vi "Save-Recall Instrument Setup from file.vi"(0 "VISA resource name":refnum<visa-resource-name>, 5 "Action (0:Save Instrument Setup)":u16(ring) items=["Save Instrument Setup", "Recall Instrument Setup"], 9 "Timeout (10000)":u32=10000, 11 "error in (no error)":errorcluster, 12 "Path":string, 13 "Filename (PANEL.SET)":string="PANEL.SET") -> (4 "VISA resource name out":refnum<visa-resource-name>, 15 "error out":errorcluster)   [LabVIEW 2021, in "Siglent SDS 1000 2000 Series.lvlib"]
doc: "Stores or recalls the current state of your instrument to/from a file on the scope's harddrive.\n\nNote:\nTo save or recall panel setups to one of the \"internal\" non-volatile memories, use the VI \"Save-Recall Setup from Device\""
uses:
  <instrlib>/Siglent SDS 1000 2000 Series/Siglent SDS 1000 2000 Series.lvlib
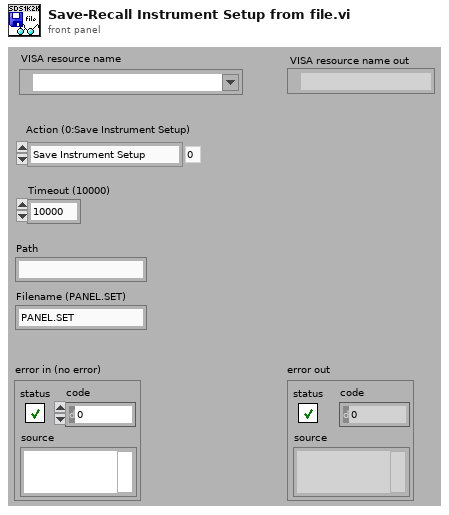
[diagram p1: front panel]
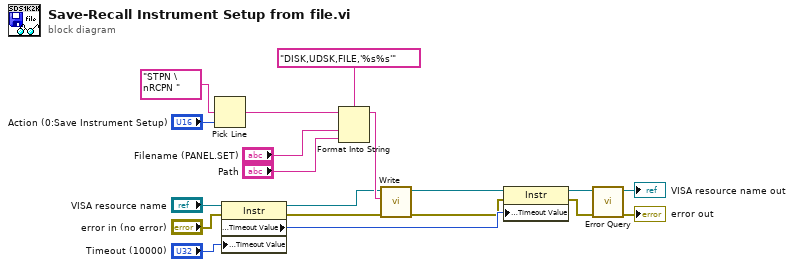
[diagram p0: block diagram]
diagram:
  n1 = Pick Line(multi-line string="STPN \nRCPN ", line index="Action (0:Save Instrument Setup)") -> (output string=w3:string)  [unwired: 1 in]
  n2 = property class="Instr"(reference="VISA resource name", error in="error in (no error)", "General Settings:Timeout Value"="Timeout (10000)") -> (reference out=w13:refnum<visa-resource-name>, error out=w8:errorcluster, "General Settings:Timeout Value"=w7:u32)
  n3 = Format Into String(format string="DISK,UDSK,FILE,'%s%s'", initial string=w3, "Filename (PANEL.SET)", "Path") -> (resulting string=w17:string)  [unwired: 1 in, 1 out]
  n4 = call <instrlib>:"Write.vi"("error in (no error)"=w8, "Write Buffer"=w17, "VISA resource name"=w13) -> ("error out"=w1:errorcluster, "VISA resource name out"=w2:refnum<visa-resource-name>)  [unwired: 6 in, 1 out]
  n5 = property class="Instr"(reference=w2, error in=w1, "General Settings:Timeout Value"=w7) -> (reference out=w12:refnum<visa-resource-name>, error out=w4:errorcluster)
  n6 = call <instrlib>:"Error Query.vi"("error in (no error)"=w4, "VISA resource name"=w12) -> ("error out"=→"error out":errorcluster, "VISA resource name out"=→"VISA resource name out":refnum<visa-resource-name>)  [unwired: 6 in, 2 out]
